vi "BuildCustomDashBoardData.vi"   [LabVIEW 2014]
doc: "This VI builds data and sends it back to the dashboard PC program. By default it sends back the raw values for the first analog, digital, and solenoid module. Modify it to send back the data you want to view. Consider adding higher level data to the Dashboard Datatype.ctl and to this VI. Then update the Dashboard to display the data however you like.\n\nThis software is licensed. Open the labview\\readme\\WPI Robotics Library Open Source License.txt file for more information."
uses:
  <vilib>/Rock Robotics/WPI/DriverStation/WPI_DriverStationRobotMode2.ctl
  typedefs/dashboard/DashboardEnable.ctl
  <vilib>/Rock Robotics/SystemInterfaces/Typedef/FPGA_TypedefDigitalModule.ctl
  typedefs/fg_getset.ctl
  <vilib>/Rock Robotics/WPI/AnalogModule/WPI_AnalogModuleDevStatus.ctl
  <vilib>/Rock Robotics/SystemInterfaces/Typedef/FPGA_TypedefAnalogModule.ctl
  <vilib>/Rock Robotics/SystemInterfaces/AI/FPGA_AIChannel.ctl
  <vilib>/Rock Robotics/WPI/Solenoid/WPI_SolenoidDevRef.ctl
  <vilib>/Rock Robotics/WPI/Solenoid/WPI_SolenoidChannel.ctl
  <vilib>/Rock Robotics/WPI/DriverStation/WPI_DriverStationDigitalData.ctl
  <vilib>/Rock Robotics/SystemInterfaces/DIO/FPGA_DIOPWMChannel.ctl
  <vilib>/Rock Robotics/Network Tables/NT Write String Array.vi
  <vilib>/Rock Robotics/WPI/Compressor/WPI_CompressorGetSetRefNum.vi
  global variables/safeties.vi
  <vilib>/Rock Robotics/WPI/Solenoid/Deprecated/WPI_SolenoidGetBool.vi
  <vilib>/Rock Robotics/SystemInterfaces/System/FPGA_SystemGet.vi
  global variables/devrefs.vi
  global variables/state machine.vi
  typedefs/dashboard/misc dash data.ctl
  typedefs/test/test controls.ctl
  global variables/vision.vi
  typedefs/state machine/performance data.ctl
panel:
  # "Generate Dashboard Data and Send it"
  # "Note: Test code calls some dashboard data, which is gotten there not here"
types:
  T1 = typedef "WPI_AnalogModuleDevStatus.ctl" = cluster{"DevStatus":errorcluster, "Controller":T2}
  T2 = typedef "FPGA_TypedefAnalogModule.ctl" = enum16{"Controller 1"}
  T3 = typedef "FPGA_AIChannel.ctl" = enum8{"AI 0", "AI 1", "AI 2", "AI 3", "AI MXP 0", "AI MXP 1", "AI MXP 2", "AI MXP 3", "Invalid"}
  T4 = typedef "FPGA_TypedefDigitalModule.ctl" = enum16{"Controller 1"}
  T5 = typedef "WPI_DriverStationDigitalData.ctl" = cluster{"Relay Fwd":u8, "Relay Rev":u8, "GPIO":u16, "GPIO_OE":u16, "PWM":cluster{"PWM[0]":u8, "PWM[1]":u8, "PWM[2]":u8, "PWM[3]":u8, "PWM[4]":u8, "PWM[5]":u8, "PWM[6]":u8, "PWM[7]":u8, "PWM[8]":u8, "PWM[9]":u8, "PWM[10]":u8, "PWM[11]":u8, "PWM[12]":u8, "PWM[13]":u8, "PWM[14]":u8, "PWM[15]":u8, "PWM[16]":u8, "PWM[17]":u8, "PWM[18]":u8, "PWM[19]":u8}}
  T6 = typedef "FPGA_DIOPWMChannel.ctl" = enum8{"PWM 0", "PWM 1", "PWM 2", "PWM 3", "PWM 4", "PWM 5", "PWM 6", "PWM 7", "PWM 8", "PWM 9", "PWM MXP 0", "PWM MXP 1", "PWM MXP 2", "PWM MXP 3", "PWM MXP 4", "PWM MXP 5", "PWM MXP 6", "PWM MXP 7", "PWM MXP 8", "PWM MXP 9", "Invalid"}
  T7 = typedef "WPI_SolenoidChannel.ctl" = enum8{"Solenoid 0", "Solenoid 1", "Solenoid 2", "Solenoid 3", "Solenoid 4", "Solenoid 5", "Solenoid 6", "Solenoid 7", "Invalid"}
  T8 = typedef "WPI_SolenoidDevRef.ctl" = cluster{"DevStatus":errorcluster, "Pneumatics Control Module":u8, "Forward Solenoid Channel":T7, "Reverse Solenoid Channel":T7}
  T9 = typedef "misc dash data.ctl" = cluster{"Performance":T10, "Vision":cluster{"distance":dbl}, "Enabled?":bool}
  T10 = typedef "performance data.ctl" = cluster{"Vision mSPI":u32, "Main mSPI":u32, "Dash mSPI":u32}
  T11 = typedef "fg_getset.ctl" = enum16{"Get", "Set"}
  T12 = typedef "WPI_DriverStationRobotMode2.ctl" = enum16{"Autonomous Disabled", "Autonomous Enabled", "Teleop Disabled", "Teleop Enabled", "Disconnected", "Finish", "Test Disabled", "Test Enabled", "Emergency Stopped"}
  T13 = typedef "DashboardEnable.ctl" = cluster{"Analog I/O":bool[], "Digital I/O":bool, "Solenoids":bool}
  T14 = typedef "subStates.ctl" = enum16{"null", "wait", "driver control", "auto", "manual override", "hold position", "rotate", "test", "end"}
  T15 = typedef "FPGA_DIODevRef.ctl" = cluster{"DevStatus":errorcluster, "Controller":T4}
  T16 = cluster{"[0]":u16, "[1]":u16, "[2]":u16, "[3]":u16, "[4]":u16, "[5]":u16, "[6]":u16, "[7]":u16, "[8]":u16, "[9]":u16}
  T17 = typedef "WPI_EncoderDevRef.ctl" = cluster{"DevStatus":errorcluster, "EncoderIndex":T18, "CounterIndex":T19, "DistancePerCount":dbl, "Decoding Type":T20}
  T18 = typedef "FPGA_EncoderIdx.ctl" = enum8{"Enc 0", "Enc 1", "Enc 2", "Enc 3", "Enc 4", "Enc 5", "Enc 6", "Enc 7", "Invalid"}
  T19 = typedef "FPGA_CounterCtrSystemIndex.ctl" = enum8{"Ctr 0", "Ctr 1", "Ctr 2", "Ctr 3", "Ctr 4", "Ctr 5", "Ctr 6", "Ctr 7", "Invalid"}
  T20 = typedef "WPI_EncoderType.ctl" = enum16{"1x", "2x", "4x"}
  T21 = typedef "WPI_CompressorDevRef.ctl" = cluster{"DevStatus":errorcluster, "Pneumatics Control Module":u8}
  T22 = typedef "WPI_MotorControlDeviceRef.ctl" = cluster{"DeviceStatus":errorcluster, "Type":T23, "PWM":cluster{"Controller":T4, "PWM Channel":T6, "DeadBand":T24}, "CAN":cluster{"Device Number":u8, "Control Mode":T25, "Semaphore":T26, "Max Vout":dbl, "TalonSRX Control Mode":T27}, "Invert":bool, "TransformRef":T28, "InvTransformRef":T28}
  T23 = typedef "WPI_MotorControlType.ctl" = enum16{"PWM", "CAN", "CANTalonSRX"}
  T24 = typedef "WPI_PWMDeadband.ctl" = cluster{"Name":string, "maxPositivePwm":i32, "minPositivePwm":i32, "centerPwm":i32, "maxNegativePwm":i32, "minNegativePwm":i32, "angularRange":u16}
  T25 = typedef "WPI_CANJaguar_ControlMode.ctl" = enum8{"Percent VBus", "Current", "Speed", "Position", "Voltage"}
  T26 = typedef "Semaphore RefNum" = refnum<k1>
  T27 = typedef "WPI_CANTalonSRX_APIControlMode.ctl" = enum8{"Percent VBus", "Speed", "Position", "Slave", "Unchanged / Invalid"}
  T28 = typedef "WPI_PWMTransform_ConPane.ctl" = refnum<vi>
  T29 = typedef "WPI_GyroDevRef.ctl" = cluster{"DevStatus":errorcluster, "Analog Module":T2, "Analog Channel":T3, "Offset":dbl, "Gain (VoltsPerDegree/Second)":dbl}
  T30 = typedef "singleUseSubstate.ctl" = enum16{"null", "wait", "extend left", "retract left", "extend right", "retract right", "end"}
  T31 = typedef "h-drive teleop safety data.ctl" = cluster{"Back Left Encoder Failure":bool, "Back Left No Rate Read":bool, "Back Right Encoder Failure":bool, "Back Right No Rate Read":bool, "Front Left Encoder Failure":bool, "Front Left No Rate Read":bool, "Front Right Encoder Failure":bool, "Front Right No Rate Read":bool, "No Gyro Rate Read":bool, "Gyro Failure":bool}
  T32 = typedef "test controls.ctl" = cluster{"Button":bool, "Switch":bool, "Slider":dbl}
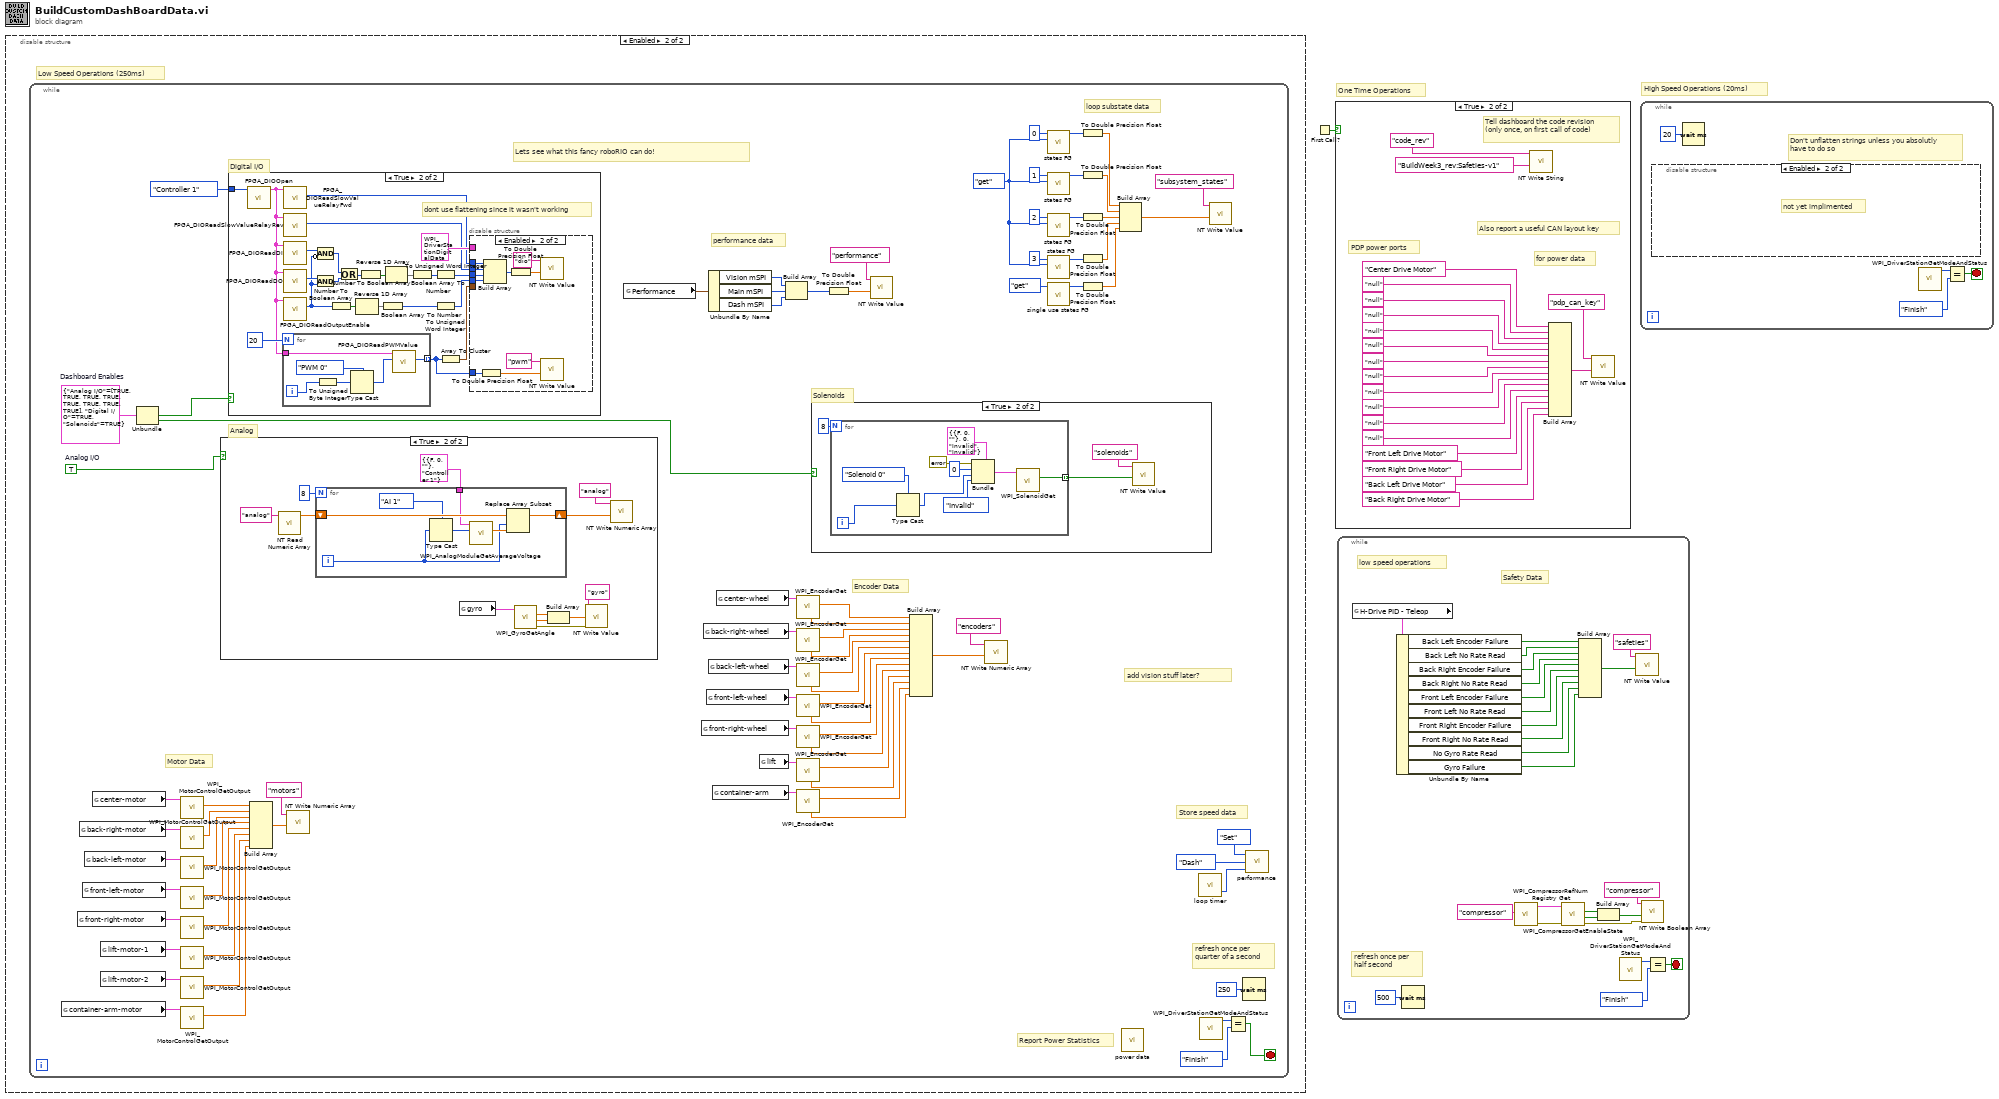
[diagram p0: block diagram]
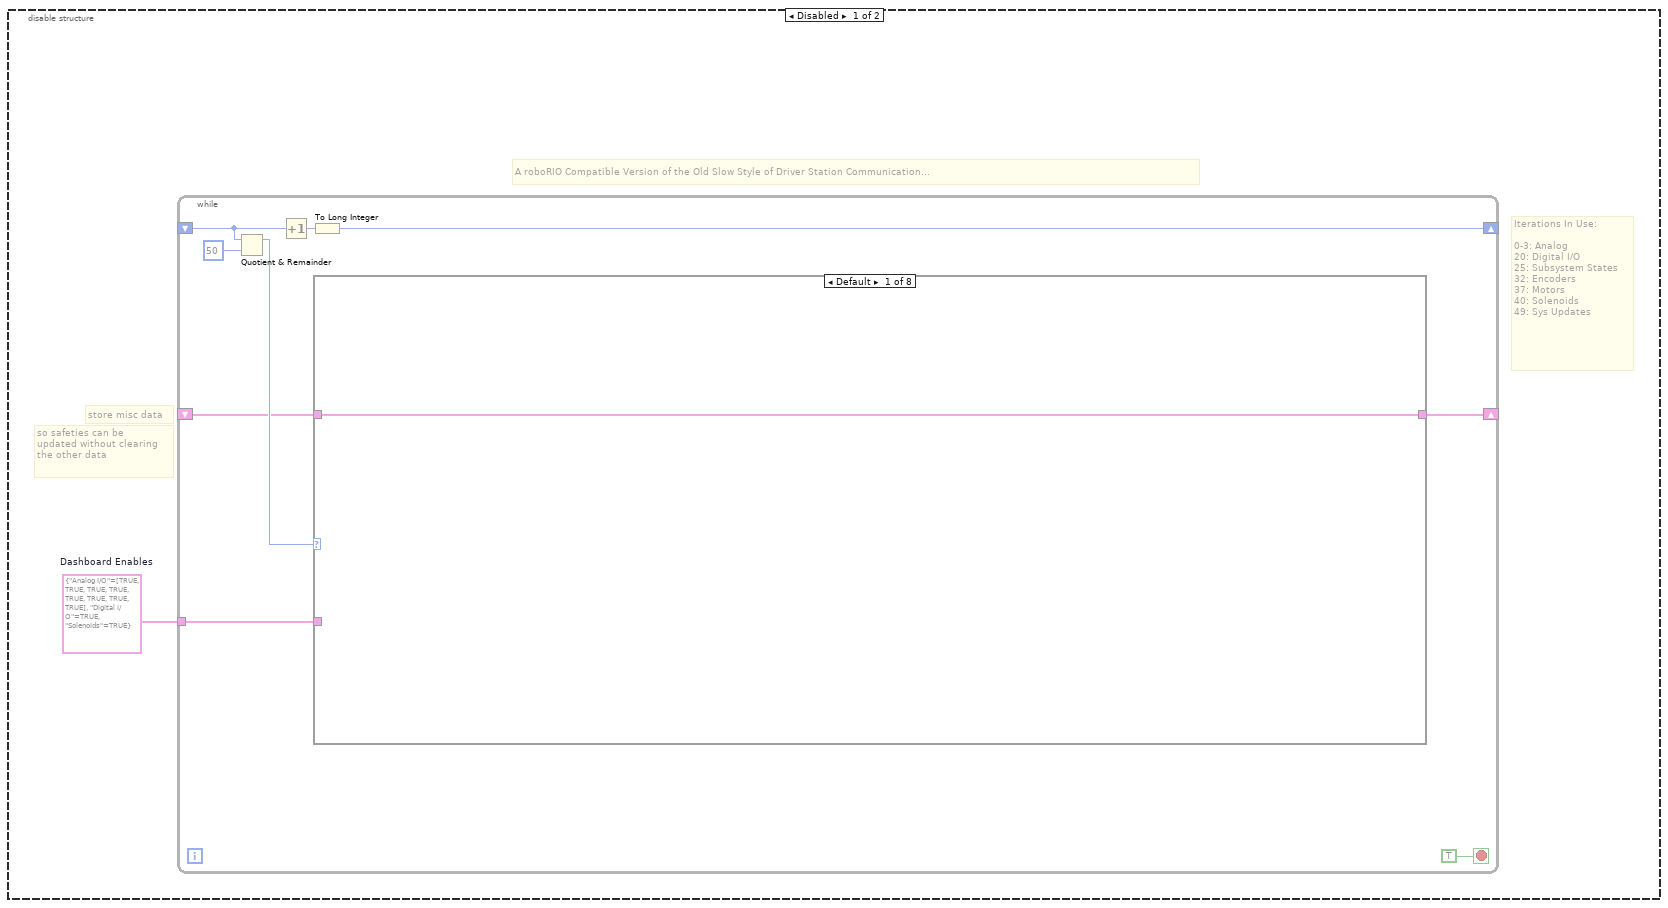
[diagram p2: hidden frame]
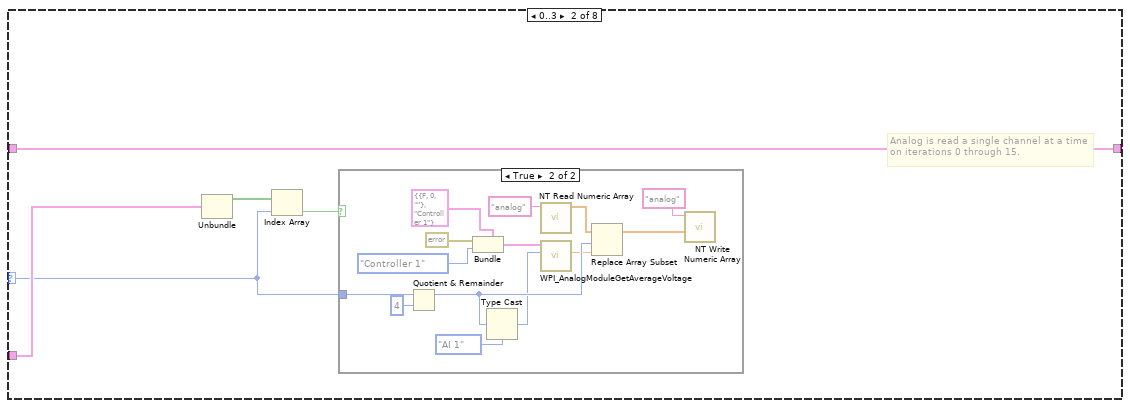
[diagram p3: hidden frame]
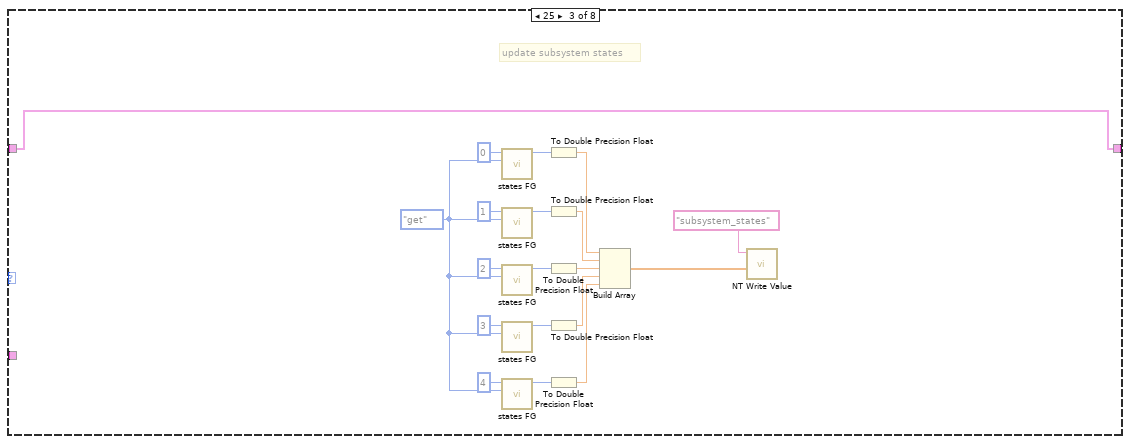
[diagram p5: hidden frame]
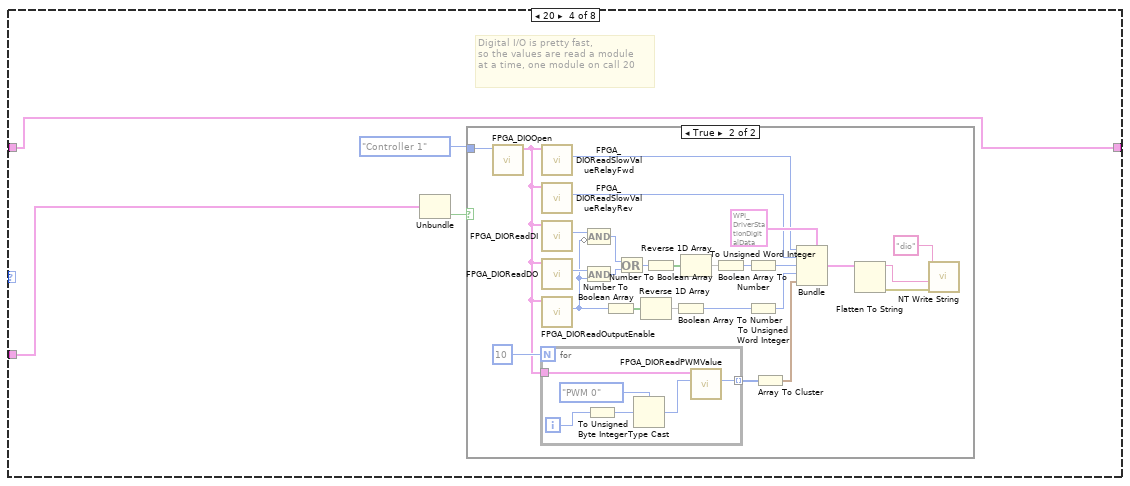
[diagram p6: hidden frame]
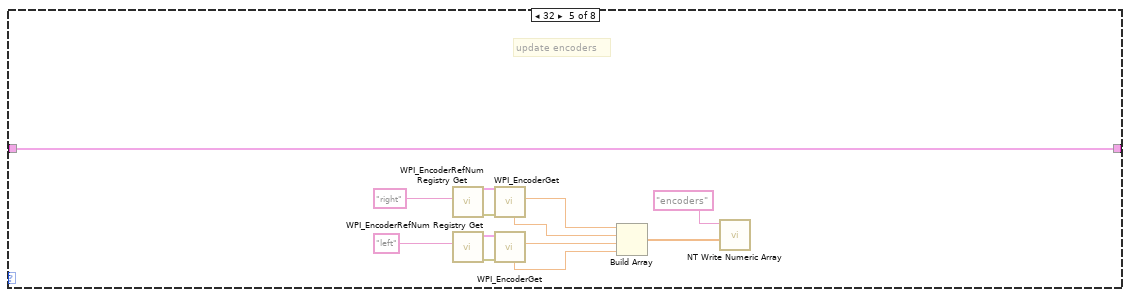
[diagram p8: hidden frame]
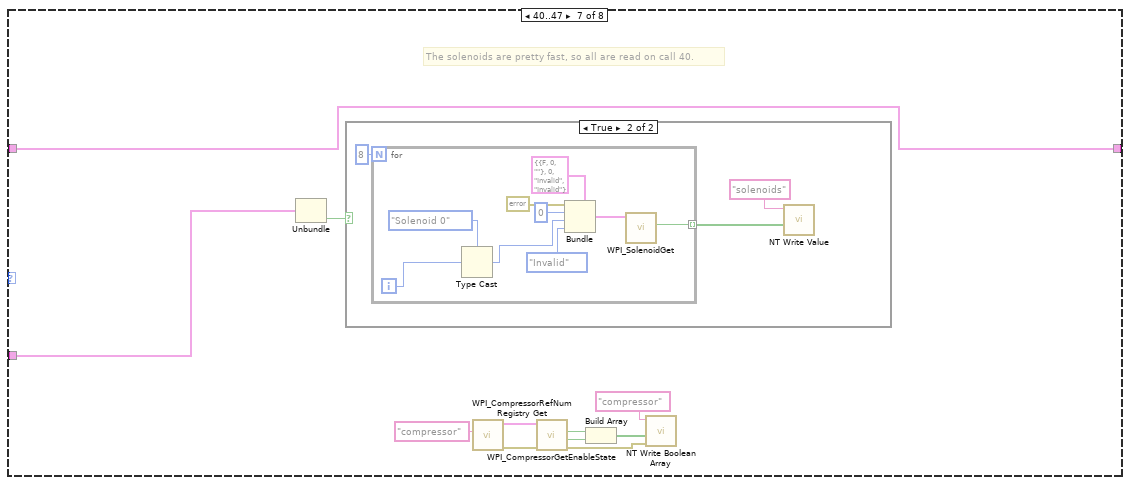
[diagram p10: hidden frame]
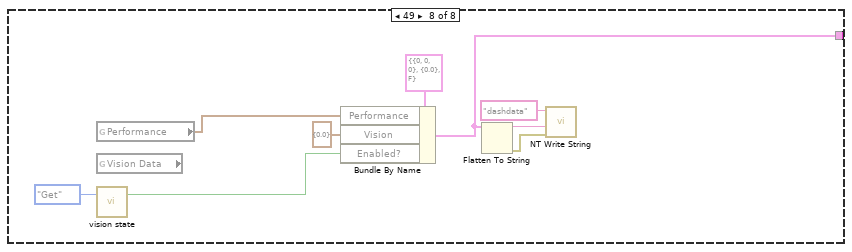
[diagram p12: hidden frame]
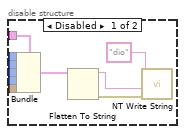
[diagram p15: hidden frame]
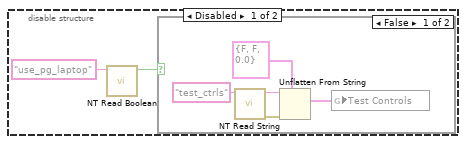
[diagram p17: hidden frame]
diagram:
  # "One Time Operations"
  # "High Speed Operations (20ms)"
  n1 = disable-structure shown="Enabled" {
    frame Disabled {
      w2 = T13 {"Analog I/O"=[TRUE, TRUE, TRUE, TRUE, TRUE, TRUE, TRUE, TRUE], "Digital I/O"=TRUE, "Solenoids"=TRUE}  # Dashboard Enables
      # "A roboRIO Compatible Version of the Old Slow Style of Driver Station Communication..."
      # "so safeties can be\nupdated without clearing\nthe other data"
      # "store misc data"
      # "Iterations In Use:\n\n0-3: Analog\n20: Digital I/O \n25: Subsystem States\n32: Encoders\n37: Motors\n40: Solenoids\n49: Sys Updates"
      n2 = while {
        shift-right: [w8] -> _
        shift-left: _ -> [w9]
        tunnel: w2 -> [w6]
        shift-right: [w4] -> _
        shift-left: _ -> [w3]
        stop <- TRUE stop-if-true
        n3 = Quotient & Remainder(x=w9, y=50) -> (x-y*floor(x/y)=w5:i32)  [unwired: 1 out]
        n4 = Increment(x=w9) -> (x+1=w10:i32)
        n5 = To Long Integer(number=w10) -> (32bit integer=w8:i32)
        n6 = case shown="Default" w5 {
          selector: w5 -> [_ w16 _ _ _ _ _ _]
          tunnel: w6 -> [_ w17 _ w54 _ _ w111 _]
          tunnel: [w12 w14 w33 w51 w89 w100 w102 w127] -> w4
          tunnel: w3 -> [w12 w14 w33 w51 w89 w100 w102 _]
          frame Default {
          }
          frame 0..3 {
            # "Analog is read a single channel at a time\non iterations 0 through 15."
            n7 = Unbundle(w17) -> ("Analog I/O"=w13:bool[])  [unwired: 2 out]
            n8 = Index Array(array=w13, index=w16) -> (element=w15:bool)
            n9 = case shown="True" w15 {
              tunnel: w16 -> [_ w29]
              frame False {
              }
              frame True {
                n10 = Quotient & Remainder(x=w29, y=4) -> (x-y*floor(x/y)=w23:i32)  [unwired: 1 out]
                n11 = Bundle(cluster=T1 {"DevStatus"={"status"=FALSE, "code"=0, "source"=""}, "Controller"=enum."Controller 1"} ("AnalogModuleDevStatus"), "DevStatus"=errorcluster {"status"=FALSE, "code"=0, "source"=""}, "Controller"=FPGA_TypedefAnalogModule."Controller 1") -> (w20:T1)
                n12 = Type Cast(type=FPGA_AIChannel."AI 1" ("Channel"), x=w23) -> (*(type *) &x=w22:T3)
                n13 = call <vilib>:"NT Read Numeric Array.vi"("Name"="analog") -> ("Numeric Array"=w27:dbl[])  [unwired: 9 in, 1 out]
                n14 = call <vilib>:"WPI_AnalogModuleGetAverageVoltage.vi"("Channel"=w22, "AnalogModuleDevStatus"=w20) -> ("Average Voltage"=w18:dbl)  [unwired: 1 in, 8 out]
                n15 = Replace Array Subset(array=w27, new element=w18, index=w23) -> (w25:dbl[])
                n16 = call <vilib>:"NT Write Numeric Array.vi"("Numeric Array"=w25, "Name"="analog") -> ()  [unwired: 9 in, 1 out]
              }
            }
          }
          frame 25 {
            w45 = enum16{"set", "get"}."get" ("menu (get)")
            # "update subsystem states"
            n17 = call "states FG.vi"("menu (get)"=w45, "Loop ID"=0) -> ("subState out"=w42:T14)  [unwired: 6 in, 3 out]
            n18 = call "states FG.vi"("menu (get)"=w45, "Loop ID"=1) -> ("subState out"=w43:T14)  [unwired: 6 in, 3 out]
            n19 = call "states FG.vi"("menu (get)"=w45, "Loop ID"=2) -> ("subState out"=w44:T14)  [unwired: 6 in, 3 out]
            n20 = call "states FG.vi"("menu (get)"=w45, "Loop ID"=3) -> ("subState out"=w41:T14)  [unwired: 6 in, 3 out]
            n21 = call "states FG.vi"("menu (get)"=w45, "Loop ID"=4) -> ("subState out"=w40:T14)  [unwired: 6 in, 3 out]
            n22 = To Double Precision Float(number=w42) -> (double precision float=w38:dbl)
            n23 = To Double Precision Float(number=w43) -> (double precision float=w37:dbl)
            n24 = To Double Precision Float(number=w44) -> (double precision float=w36:dbl)
            n25 = To Double Precision Float(number=w41) -> (double precision float=w35:dbl)
            n26 = To Double Precision Float(number=w40) -> (double precision float=w34:dbl)
            n27 = Build Array(w38, w37, w36, w35, w34) -> (w32:dbl[])
            n28 = call-poly <vilib>:"NT Write Value.vi"("Numeric Array"=w32, "Name"="subsystem_states") -> ()  [unwired: 9 in, 1 out]
          }
          frame 20 {
            # "Digital I/O is pretty fast,\nso the values are read a module\nat a time, one module on call 20"
            n29 = Unbundle(w54) -> ("Solenoids"=w52:bool)  [unwired: 2 out]
            n30 = case shown="True" w52 {
              tunnel: FPGA_TypedefDigitalModule."Controller 1" ("Module (Module 1)") -> [_ w61]
              frame False {
              }
              frame True {
                n31 = call <vilib>:"FPGA_DIOOpen.vi"("Controller"=w61) -> ("DIODeviceRef"=w77:T15)  [unwired: 1 in, 9 out]
                n32 = for {
                  N: 10 -> [_]
                  tunnel: w77 -> [w86]
                  tunnel: [w84] -> w78 mode=indexing
                  i -> [w85]
                  n33 = To Unsigned Byte Integer(number=w85) -> (unsigned 8bit integer=w83:u8)
                  n34 = Type Cast(type=FPGA_DIOPWMChannel."PWM 0" ("PWMChannel"), x=w83) -> (*(type *) &x=w81:T6)
                  n35 = call <vilib>:"FPGA_DIOReadPWMValue.vi"("PWMChannel"=w81, "DIODeviceRef In"=w86) -> ("PWMValue"=w84:u16)  [unwired: 1 in, 8 out]
                }
                n36 = call <vilib>:"FPGA_DIOReadSlowValueRelayFwd.vi"("DIODeviceRef In"=w77) -> ("Relay Forward"=w70:u8)  [unwired: 1 in, 9 out]
                n37 = call <vilib>:"FPGA_DIOReadSlowValueRelayRev.vi"("DIODeviceRef In"=w77) -> ("Relay Reverse"=w71:u8)  [unwired: 1 in, 9 out]
                n38 = call <vilib>:"FPGA_DIOReadDI.vi"("DIODeviceRef In"=w77) -> ("DI"=w75:u32)  [unwired: 1 in, 9 out]
                n39 = call <vilib>:"FPGA_DIOReadDO.vi"("DIODeviceRef In"=w77) -> ("DO"=w74:u32)  [unwired: 1 in, 9 out]
                n40 = call <vilib>:"FPGA_DIOReadOutputEnable.vi"("DIODeviceRef In"=w77) -> ("OutputEnable"=w65:u32)  [unwired: 1 in, 9 out]
                n41 = And(x=w74, y=w65) -> (x .and. y?=w73:u32)
                n42 = Compound Arithmetic op=AND(w75, invert w65) -> (w72:u32)
                n43 = Number To Boolean Array(number=w65) -> (Boolean array=w67:bool[])
                n44 = Or(x=w72, y=w73) -> (x .or. y?=w63:u32)
                n45 = Reverse 1D Array(array=w67) -> (reversed array=w66:bool[])
                n46 = Number To Boolean Array(number=w63) -> (Boolean array=w68:bool[])
                n47 = Boolean Array To Number(Boolean array=w66) -> (number=w64:u32)
                n48 = Reverse 1D Array(array=w68) -> (reversed array=w69:bool[])
                n49 = Boolean Array To Number(Boolean array=w69) -> (number=w62:u32)
                n50 = To Unsigned Word Integer(number=w62) -> (unsigned 16bit integer=w55:u16)
                n51 = To Unsigned Word Integer(number=w64) -> (unsigned 16bit integer=w56:u16)
                n52 = Array To Cluster(array=w78) -> (cluster=w76:T16)
                n53 = Bundle(cluster=T5 {"Relay Fwd"=0, "Relay Rev"=0, "GPIO"=0, "GPIO_OE"=0, "PWM"={"PWM[0]"=0, "PWM[1]"=0, "PWM[2]"=0, "PWM[3]"=0, "PWM[4]"=0, "PWM[5]"=0, "PWM[6]"=0, "PWM[7]"=0, "PWM[8]"=0, "PWM[9]"=0, "PWM[10]"=0, "PWM[11]"=0, "PWM[12]"=0, "PWM[13]"=0, "PWM[14]"=0, "PWM[15]"=0, "PWM[16]"=0, "PWM[17]"=0, "PWM[18]"=0, "PWM[19]"=0}} ("DigitalModule"), "Relay Fwd"=w70, "Relay Rev"=w71, "GPIO"=w55, "GPIO_OE"=w56, "PWM"=w76) -> (w60:T5)
                n54 = Flatten To String(anything=w60) -> (data string=w58:string, error out=w59:errorcluster)  [unwired: 1 in, 3 out]
                n55 = call <vilib>:"NT Write String.vi"("error in"=w59, "String"=w58, "Name"="dio") -> ()  [unwired: 8 in, 1 out]
              }
            }
          }
          frame 32 {
            # "update encoders"
            n56 = call <vilib>:"WPI_EncoderRefNum Registry Get.vi"("refnum name"="right") -> ("error out"=w97:errorcluster, "EncoderDevRef"=w96:T17)  [unwired: 9 in]
            n57 = call <vilib>:"WPI_EncoderRefNum Registry Get.vi"("refnum name"="left") -> ("error out"=w94:errorcluster, "EncoderDevRef"=w95:T17)  [unwired: 9 in]
            n58 = call <vilib>:"WPI_EncoderGet.vi"("error in (no error)"=w97, "EncoderDevRef"=w96) -> ("Distance"=w93:dbl, "Rate"=w88:dbl)  [unwired: 4 in, 4 out]
            n59 = call <vilib>:"WPI_EncoderGet.vi"("error in (no error)"=w94, "EncoderDevRef"=w95) -> ("Distance"=w92:dbl, "Rate"=w91:dbl)  [unwired: 4 in, 4 out]
            n60 = Build Array(w93, w88, w92, w91) -> (w90:dbl[])
            n61 = call <vilib>:"NT Write Numeric Array.vi"("Numeric Array"=w90, "Name"="encoders") -> ()  [unwired: 9 in, 1 out]
          }
          frame 37 {
            # "update motor array"
          }
          frame 40..47 {
            # "The solenoids are pretty fast, so all are read on call 40."
            n62 = Unbundle(w111) -> ("Solenoids"=w101:bool)  [unwired: 2 out]
            n63 = case shown="True" w101 {
              frame False {
              }
              frame True {
                n64 = for {
                  N: 8 -> [_]
                  tunnel: [w115] -> w113 mode=indexing
                  i -> [w117]
                  n65 = Type Cast(type=WPI_SolenoidChannel."Solenoid 0" ("Forward Solenoid Channel"), x=w117) -> (*(type *) &x=w116:T7)
                  n66 = Bundle(cluster=T8 {"DevStatus"={"status"=FALSE, "code"=0, "source"=""}, "Pneumatics Control Module"=0, "Forward Solenoid Channel"=enum."Invalid", "Reverse Solenoid Channel"=enum."Invalid"} ("SolenoidDevRef"), "DevStatus"=errorcluster {"status"=FALSE, "code"=0, "source"=""}, "Pneumatics Control Module"=u8 0, "Forward Solenoid Channel"=w116, "Reverse Solenoid Channel"=WPI_SolenoidChannel."Invalid") -> (w122:T8)
                  n67 = call-poly <vilib>:"WPI_SolenoidGet.vi"("SolenoidDevRef"=w122) -> ("Value"=w115:bool)  [unwired: 8 in, 2 out]
                }
                n68 = call-poly <vilib>:"NT Write Value.vi"("Boolean Array"=w113, "Name"="solenoids") -> ()  [unwired: 9 in, 1 out]
              }
            }
            n69 = call <vilib>:"WPI_CompressorRefNum Registry Get.vi"("refnum name"="compressor") -> ("error out"=w107:errorcluster, "CompressorDevRef"=w108:T21)  [unwired: 9 in]
            n70 = call <vilib>:"WPI_CompressorGetEnableState.vi"("error in (no error)"=w107, "CompressorDevRef"=w108) -> ("error out"=w103:errorcluster, "Compressor Running"=w105:bool, "Enabled"=w106:bool)  [unwired: 6 in, 1 out]
            n71 = Build Array(w106, w105) -> (w104:bool[])
            n72 = call <vilib>:"NT Write Boolean Array.vi"("error in"=w103, "Boolean Array"=w104, "Name"="compressor") -> ()  [unwired: 8 in, 1 out]
          }
          frame 49 {
            n73 = global read "state machine.vi" "Performance"() -> (w124:T10)
            n74 = global read "vision.vi" "Vision Data"() -> ()  [unwired: 1 out]
            n75 = call "vision state.vi"("Menu"=fg_getset."Get") -> ("Enabled?"=w126:bool)  [unwired: 1 in, 1 out]
            n76 = Bundle By Name(cluster=T9 {"Performance"={"Vision mSPI"=0, "Main mSPI"=0, "Dash mSPI"=0}, "Vision"={"distance"=0.0}, "Enabled?"=FALSE}, "Performance"=w124, "Vision"=cluster{"distance":dbl} {"distance"=0.0}, "Enabled?"=w126) -> (w127:T9)
            n77 = Flatten To String(anything=w127) -> (data string=w130:string, error out=w128:errorcluster)  [unwired: 1 in, 3 out]
            n78 = call <vilib>:"NT Write String.vi"("error in"=w128, "String"=w130, "Name"="dashdata") -> ()  [unwired: 8 in, 1 out]
          }
        }
      }
    }
    frame Enabled {
      # "Low Speed Operations (250ms)"
      n79 = while {
        stop <- w191 stop-if-true
        w182 = TRUE  # Analog I/O
        w205 = enum16{"set", "get"}."get" ("menu (get)")
        w210 = T13 {"Analog I/O"=[TRUE, TRUE, TRUE, TRUE, TRUE, TRUE, TRUE, TRUE], "Digital I/O"=TRUE, "Solenoids"=TRUE}  # Dashboard Enables
        # "Encoder Data"
        # "Motor Data"
        # "loop substate data"
        # "performance data"
        # "add vision stuff later?"
        # "Report Power Statistics"
        # "Store speed data"
        # "refresh once per\nquarter of a second"
        # "Solenoids"
        # "Digital I/O"
        # "Analog"
        # "Lets see what this fancy roboRIO can do!"
        n80 = global read "devrefs.vi" "container-arm-motor"() -> (w150:T22)
        n81 = global read "devrefs.vi" "front-right-motor"() -> (w154:T22)
        n82 = global read "devrefs.vi" "back-right-motor"() -> (w157:T22)
        n83 = global read "devrefs.vi" "front-left-motor"() -> (w155:T22)
        n84 = global read "devrefs.vi" "back-left-motor"() -> (w156:T22)
        n85 = global read "devrefs.vi" "center-motor"() -> (w153:T22)
        n86 = global read "devrefs.vi" "lift-motor-1"() -> (w152:T22)
        n87 = global read "devrefs.vi" "lift-motor-2"() -> (w151:T22)
        n88 = Unbundle(w210) -> ("Digital I/O"=w195:bool, "Solenoids"=w181:bool)  [unwired: 1 out]
        n89 = call <vilib>:"WPI_MotorControlGetOutput.vi"("MotorControlDevRef"=w153) -> ("Output"=w149:dbl)  [unwired: 8 in, 2 out]
        n90 = call <vilib>:"WPI_MotorControlGetOutput.vi"("MotorControlDevRef"=w157) -> ("Output"=w148:dbl)  [unwired: 8 in, 2 out]
        n91 = call <vilib>:"WPI_MotorControlGetOutput.vi"("MotorControlDevRef"=w156) -> ("Output"=w147:dbl)  [unwired: 8 in, 2 out]
        n92 = call <vilib>:"WPI_MotorControlGetOutput.vi"("MotorControlDevRef"=w155) -> ("Output"=w146:dbl)  [unwired: 8 in, 2 out]
        n93 = call <vilib>:"WPI_MotorControlGetOutput.vi"("MotorControlDevRef"=w154) -> ("Output"=w145:dbl)  [unwired: 8 in, 2 out]
        n94 = call <vilib>:"WPI_MotorControlGetOutput.vi"("MotorControlDevRef"=w152) -> ("Output"=w144:dbl)  [unwired: 8 in, 2 out]
        n95 = call <vilib>:"WPI_MotorControlGetOutput.vi"("MotorControlDevRef"=w151) -> ("Output"=w143:dbl)  [unwired: 8 in, 2 out]
        n96 = call <vilib>:"WPI_MotorControlGetOutput.vi"("MotorControlDevRef"=w150) -> ("Output"=w142:dbl)  [unwired: 8 in, 2 out]
        n97 = case shown="True" w182 {
          frame False {
          }
          frame True {
            n98 = call <vilib>:"NT Read Numeric Array.vi"("Name"="analog") -> ("Numeric Array"=w281:dbl[])  [unwired: 9 in, 1 out]
            n99 = for {
              N: 8 -> [_]
              tunnel: T1 {"DevStatus"={"status"=FALSE, "code"=0, "source"=""}, "Controller"=enum."Controller 1"} ("AnalogModuleDevStatus") -> [w284]
              shift-right: [w288] -> w280
              shift-left: w281 -> [w289]
              i -> [w283]
              n100 = Type Cast(type=FPGA_AIChannel."AI 1" ("Channel"), x=w283) -> (*(type *) &x=w286:T3)
              n101 = call <vilib>:"WPI_AnalogModuleGetAverageVoltage.vi"("Channel"=w286, "AnalogModuleDevStatus"=w284) -> ("Average Voltage"=w285:dbl)  [unwired: 1 in, 8 out]
              n102 = Replace Array Subset(array=w289, new element=w285, index=w283) -> (w288:dbl[])
            }
            n103 = global read "devrefs.vi" "gyro"() -> (w275:T29)
            n104 = call <vilib>:"WPI_GyroGetAngle.vi"("GyroDevRef"=w275) -> ("error out"=w276:errorcluster, "Angular Rate"=w273:dbl, "Angle"=w274:dbl)  [unwired: 7 in, 1 out]
            n105 = Build Array(w274, w273) -> (w272:dbl[])
            n106 = call-poly <vilib>:"NT Write Value.vi"("error in"=w276, "Numeric Array"=w272, "Name"="gyro") -> ()  [unwired: 8 in, 1 out]
            n107 = call <vilib>:"NT Write Numeric Array.vi"("Numeric Array"=w280, "Name"="analog") -> ()  [unwired: 9 in, 1 out]
          }
        }
        n108 = case shown="True" w195 {
          tunnel: FPGA_TypedefDigitalModule."Controller 1" ("Module (Module 1)") -> [_ w226]
          frame False {
          }
          frame True {
            # "dont use flattening since it wasn't working"
            n109 = call <vilib>:"FPGA_DIOOpen.vi"("Controller"=w226) -> ("DIODeviceRef"=w242:T15)  [unwired: 1 in, 9 out]
            n110 = for {
              N: 20 -> [_]
              tunnel: w242 -> [w270]
              tunnel: [w268] -> w223 mode=indexing
              i -> [w269]
              n111 = To Unsigned Byte Integer(number=w269) -> (unsigned 8bit integer=w267:u8)
              n112 = Type Cast(type=FPGA_DIOPWMChannel."PWM 0" ("PWMChannel"), x=w267) -> (*(type *) &x=w265:T6)
              n113 = call <vilib>:"FPGA_DIOReadPWMValue.vi"("PWMChannel"=w265, "DIODeviceRef In"=w270) -> ("PWMValue"=w268:u16)  [unwired: 1 in, 8 out]
            }
            n114 = call <vilib>:"FPGA_DIOReadSlowValueRelayFwd.vi"("DIODeviceRef In"=w242) -> ("Relay Forward"=w235:u8)  [unwired: 1 in, 9 out]
            n115 = call <vilib>:"FPGA_DIOReadSlowValueRelayRev.vi"("DIODeviceRef In"=w242) -> ("Relay Reverse"=w236:u8)  [unwired: 1 in, 9 out]
            n116 = call <vilib>:"FPGA_DIOReadDI.vi"("DIODeviceRef In"=w242) -> ("DI"=w240:u32)  [unwired: 1 in, 9 out]
            n117 = call <vilib>:"FPGA_DIOReadDO.vi"("DIODeviceRef In"=w242) -> ("DO"=w239:u32)  [unwired: 1 in, 9 out]
            n118 = call <vilib>:"FPGA_DIOReadOutputEnable.vi"("DIODeviceRef In"=w242) -> ("OutputEnable"=w230:u32)  [unwired: 1 in, 9 out]
            n119 = And(x=w239, y=w230) -> (x .and. y?=w238:u32)
            n120 = Compound Arithmetic op=AND(w240, invert w230) -> (w237:u32)
            n121 = Number To Boolean Array(number=w230) -> (Boolean array=w232:bool[])
            n122 = Or(x=w237, y=w238) -> (x .or. y?=w228:u32)
            n123 = Reverse 1D Array(array=w232) -> (reversed array=w231:bool[])
            n124 = Number To Boolean Array(number=w228) -> (Boolean array=w233:bool[])
            n125 = Boolean Array To Number(Boolean array=w231) -> (number=w229:u32)
            n126 = Reverse 1D Array(array=w233) -> (reversed array=w234:bool[])
            n127 = Boolean Array To Number(Boolean array=w234) -> (number=w227:u32)
            n128 = To Unsigned Word Integer(number=w227) -> (unsigned 16bit integer=w224:u16)
            n129 = To Unsigned Word Integer(number=w229) -> (unsigned 16bit integer=w225:u16)
            n130 = Array To Cluster(array=w223) -> (cluster=w241:T16)
            n131 = disable-structure shown="Enabled" {
              disable-tunnel: T5 {"Relay Fwd"=0, "Relay Rev"=0, "GPIO"=0, "GPIO_OE"=0, "PWM"={"PWM[0]"=0, "PWM[1]"=0, "PWM[2]"=0, "PWM[3]"=0, "PWM[4]"=0, "PWM[5]"=0, "PWM[6]"=0, "PWM[7]"=0, "PWM[8]"=0, "PWM[9]"=0, "PWM[10]"=0, "PWM[11]"=0, "PWM[12]"=0, "PWM[13]"=0, "PWM[14]"=0, "PWM[15]"=0, "PWM[16]"=0, "PWM[17]"=0, "PWM[18]"=0, "PWM[19]"=0}} ("DigitalModule") -> [w254 _]
              disable-tunnel: w241 -> [w253 _]
              disable-tunnel: w236 -> [w252 w259]
              disable-tunnel: w235 -> [w251 w260]
              disable-tunnel: w225 -> [w246 w257]
              disable-tunnel: w224 -> [w245 w258]
              disable-tunnel: w223 -> [_ w263]
              frame Disabled {
                n132 = Bundle(cluster=w254, "Relay Fwd"=w251, "Relay Rev"=w252, "GPIO"=w245, "GPIO_OE"=w246, "PWM"=w253) -> (w250:T5)
                n133 = Flatten To String(anything=w250) -> (data string=w248:string, error out=w249:errorcluster)  [unwired: 1 in, 3 out]
                n134 = call <vilib>:"NT Write String.vi"("error in"=w249, "String"=w248, "Name"="dio") -> ()  [unwired: 8 in, 1 out]
              }
              frame Enabled {
                n135 = To Double Precision Float(number=w263) -> (double precision float=w262:dbl[])
                n136 = Build Array(w260, w259, w258, w257) -> (w256:u16[])
                n137 = To Double Precision Float(number=w256) -> (double precision float=w255:dbl[])
                n138 = call-poly <vilib>:"NT Write Value.vi"("Numeric Array"=w255, "Name"="dio") -> ()  [unwired: 9 in, 1 out]
                n139 = call-poly <vilib>:"NT Write Value.vi"("Numeric Array"=w262, "Name"="pwm") -> ()  [unwired: 9 in, 1 out]
              }
            }
          }
        }
        n140 = Build Array(w149, w148, w147, w146, w145, w144, w143, w142) -> (w140:dbl[])
        n141 = call <vilib>:"NT Write Numeric Array.vi"("Numeric Array"=w140, "Name"="motors") -> ()  [unwired: 9 in, 1 out]
        n142 = global read "state machine.vi" "Performance"() -> (w139:T10)
        n143 = global read "devrefs.vi" "front-right-wheel"() -> (w160:T17)
        n144 = global read "devrefs.vi" "back-right-wheel"() -> (w163:T17)
        n145 = global read "devrefs.vi" "front-left-wheel"() -> (w161:T17)
        n146 = Unbundle By Name(w139) -> ("Vision mSPI"=w138:u32, "Main mSPI"=w137:u32, "Dash mSPI"=w136:u32)
        n147 = global read "devrefs.vi" "back-left-wheel"() -> (w162:T17)
        n148 = global read "devrefs.vi" "container-arm"() -> (w158:T17)
        n149 = global read "devrefs.vi" "center-wheel"() -> (w164:T17)
        n150 = global read "devrefs.vi" "lift"() -> (w159:T17)
        n151 = Build Array(w138, w137, w136) -> (w135:u32[])
        n152 = call <vilib>:"WPI_EncoderGet.vi"("EncoderDevRef"=w164) -> ("Distance"=w180:dbl, "Rate"=w176:dbl)  [unwired: 5 in, 4 out]
        n153 = call <vilib>:"WPI_EncoderGet.vi"("EncoderDevRef"=w163) -> ("Distance"=w179:dbl, "Rate"=w178:dbl)  [unwired: 5 in, 4 out]
        n154 = call <vilib>:"WPI_EncoderGet.vi"("EncoderDevRef"=w162) -> ("Distance"=w174:dbl, "Rate"=w173:dbl)  [unwired: 5 in, 4 out]
        n155 = call <vilib>:"WPI_EncoderGet.vi"("EncoderDevRef"=w161) -> ("Distance"=w172:dbl, "Rate"=w171:dbl)  [unwired: 5 in, 4 out]
        n156 = call <vilib>:"WPI_EncoderGet.vi"("EncoderDevRef"=w160) -> ("Distance"=w170:dbl, "Rate"=w169:dbl)  [unwired: 5 in, 4 out]
        n157 = call <vilib>:"WPI_EncoderGet.vi"("EncoderDevRef"=w159) -> ("Distance"=w168:dbl, "Rate"=w167:dbl)  [unwired: 5 in, 4 out]
        n158 = call <vilib>:"WPI_EncoderGet.vi"("EncoderDevRef"=w158) -> ("Distance"=w166:dbl, "Rate"=w165:dbl)  [unwired: 5 in, 4 out]
        n159 = case shown="True" w181 {
          frame False {
          }
          frame True {
            n160 = for {
              N: 8 -> [_]
              tunnel: [w214] -> w212 mode=indexing
              i -> [w216]
              n161 = Type Cast(type=WPI_SolenoidChannel."Solenoid 0" ("Forward Solenoid Channel"), x=w216) -> (*(type *) &x=w215:T7)
              n162 = Bundle(cluster=T8 {"DevStatus"={"status"=FALSE, "code"=0, "source"=""}, "Pneumatics Control Module"=0, "Forward Solenoid Channel"=enum."Invalid", "Reverse Solenoid Channel"=enum."Invalid"} ("SolenoidDevRef"), "DevStatus"=errorcluster {"status"=FALSE, "code"=0, "source"=""}, "Pneumatics Control Module"=u8 0, "Forward Solenoid Channel"=w215, "Reverse Solenoid Channel"=WPI_SolenoidChannel."Invalid") -> (w221:T8)
              n163 = call-poly <vilib>:"WPI_SolenoidGet.vi"("SolenoidDevRef"=w221) -> ("Value"=w214:bool)  [unwired: 8 in, 2 out]
            }
            n164 = call-poly <vilib>:"NT Write Value.vi"("Boolean Array"=w212, "Name"="solenoids") -> ()  [unwired: 9 in, 1 out]
          }
        }
        n165 = To Double Precision Float(number=w135) -> (double precision float=w134:dbl[])
        n166 = call-poly <vilib>:"NT Write Value.vi"("Numeric Array"=w134, "Name"="performance") -> ()  [unwired: 9 in, 1 out]
        n167 = Build Array(w180, w176, w179, w178, w174, w173, w172, w171, w170, w169, w168, w167, w166, w165) -> (w177:dbl[])
        n168 = call <vilib>:"NT Write Numeric Array.vi"("Numeric Array"=w177, "Name"="encoders") -> ()  [unwired: 9 in, 1 out]
        n169 = call "states FG.vi"("menu (get)"=w205, "Loop ID"=0) -> ("subState out"=w202:T14)  [unwired: 6 in, 3 out]
        n170 = call "states FG.vi"("menu (get)"=w205, "Loop ID"=1) -> ("subState out"=w203:T14)  [unwired: 6 in, 3 out]
        n171 = call "states FG.vi"("menu (get)"=w205, "Loop ID"=2) -> ("subState out"=w204:T14)  [unwired: 6 in, 3 out]
        n172 = call "states FG.vi"("menu (get)"=w205, "Loop ID"=3) -> ("subState out"=w201:T14)  [unwired: 6 in, 3 out]
        n173 = call "single use states FG.vi"("menu (get)"=enum16{"set", "get"}."get") -> ("substate out"=w183:T30)  [unwired: 7 in, 3 out]
        n174 = To Double Precision Float(number=w202) -> (double precision float=w199:dbl)
        n175 = To Double Precision Float(number=w203) -> (double precision float=w198:dbl)
        n176 = To Double Precision Float(number=w204) -> (double precision float=w197:dbl)
        n177 = To Double Precision Float(number=w201) -> (double precision float=w185:dbl)
        n178 = To Double Precision Float(number=w183) -> (double precision float=w184:dbl)
        n179 = Build Array(w199, w198, w197, w185, w184) -> (w187:dbl[])
        n180 = call "power data.vi"() -> ()  [unwired: 12 in]
        n181 = call "loop timer.vi"() -> ("mSPI"=w188:u32)  [unwired: 1 in, 1 out]
        n182 = call <vilib>:"WPI_DriverStationGetModeAndStatus.vi"() -> ("Robot Mode"=w193:T12)  [unwired: 10 in, 1 out]
        n183 = call-poly <vilib>:"NT Write Value.vi"("Numeric Array"=w187, "Name"="subsystem_states") -> ()  [unwired: 9 in, 1 out]
        n184 = Equal?(x=w193, y=WPI_DriverStationRobotMode2."Finish") -> (x = y?=w191:bool)
        n185 = Wait (ms)(milliseconds to wait=u32 250) -> ()  [unwired: 1 out]
        n186 = call "performance.vi"("mSPI"=w188, "Loop"=enum16{"Vision", "Main", "Dash"}."Dash", "Menu"=fg_getset."Set") -> ()  [unwired: 1 out]
      }
    }
  }
  n187 = First Call?() -> (First Call?: T/F=w1:bool)
  n188 = case shown="True" w1 {
    frame False {
    }
    frame True {
      # "PDP power ports"
      # "Also report a useful CAN layout key"
      # "Tell dashboard the code revision \n(only once, on first call of code)"
      # "for power data"
      n189 = call <vilib>:"NT Write String.vi"("String"="BuildWeek3_rev:Safeties-v1", "Name"="code_rev") -> ()  [unwired: 9 in, 1 out]
      n190 = Build Array("Center Drive Motor", "null", "null", "null", "null", "null", "null", "null", "null", "null", "null", "null", "Front Left Drive Motor", "Front Right Drive Motor", "Back Left Drive Motor", "Back Right Drive Motor") -> (w302:string[])
      n191 = call-poly <vilib>:"NT Write Value.vi"("String Array"=w302, "Name"="pdp_can_key") -> ()  [unwired: 9 in, 1 out]
    }
  }
  n192 = while {
    stop <- w321 stop-if-true
    # "refresh once per\nhalf second"
    # "Safety Data"
    # "low speed operations"
    n193 = global read "safeties.vi" "H-Drive PID - Teleop"() -> (w320:T31)
    n194 = Unbundle By Name(w320) -> ("Back Left Encoder Failure"=w319:bool, "Back Left No Rate Read"=w318:bool, "Back Right Encoder Failure"=w317:bool, "Back Right No Rate Read"=w316:bool, "Front Left Encoder Failure"=w315:bool, "Front Left No Rate Read"=w314:bool, "Front Right Encoder Failure"=w313:bool, "Front Right No Rate Read"=w312:bool, "No Gyro Rate Read"=w311:bool, "Gyro Failure"=w310:bool)
    n195 = Wait (ms)(milliseconds to wait=u32 500) -> ()  [unwired: 1 out]
    n196 = call <vilib>:"WPI_CompressorRefNum Registry Get.vi"("refnum name"="compressor") -> ("error out"=w329:errorcluster, "CompressorDevRef"=w330:T21)  [unwired: 9 in]
    n197 = call <vilib>:"WPI_CompressorGetEnableState.vi"("error in (no error)"=w329, "CompressorDevRef"=w330) -> ("error out"=w325:errorcluster, "Compressor Running"=w327:bool, "Enabled"=w328:bool)  [unwired: 6 in, 1 out]
    n198 = Build Array(w319, w318, w317, w316, w315, w314, w313, w312, w311, w310) -> (w334:bool[])
    n199 = Build Array(w328, w327) -> (w326:bool[])
    n200 = call <vilib>:"WPI_DriverStationGetModeAndStatus.vi"() -> ("Robot Mode"=w322:T12)  [unwired: 10 in, 1 out]
    n201 = call-poly <vilib>:"NT Write Value.vi"("Boolean Array"=w334, "Name"="safeties") -> ()  [unwired: 9 in, 1 out]
    n202 = call <vilib>:"NT Write Boolean Array.vi"("error in"=w325, "Boolean Array"=w326, "Name"="compressor") -> ()  [unwired: 8 in, 1 out]
    n203 = Equal?(x=w322, y=WPI_DriverStationRobotMode2."Finish") -> (x = y?=w321:bool)
  }
  n204 = while {
    stop <- w336 stop-if-true
    # "Don't unflatten strings unless you absolutly\nhave to do so"
    n205 = disable-structure shown="Enabled" {
      frame Disabled {
        n206 = call <vilib>:"NT Read Boolean.vi"("Name"="use_pg_laptop") -> ("Boolean"=w340:bool)  [unwired: 9 in, 1 out]
        n207 = case shown="False" w340 {
          frame False {
            n208 = call <vilib>:"NT Read String.vi"("Name"="test_ctrls") -> ("error out"=w344:errorcluster, "String"=w343:string)  [unwired: 9 in]
            n209 = Unflatten From String(type=T32 {"Button"=FALSE, "Switch"=FALSE, "Slider"=0.0} ("Test Controls"), binary string=w343, error in (no error)=w344) -> (value=w341:T32)  [unwired: 2 in, 2 out]
            n210 = global write "state machine.vi" "Test Controls"(w341) -> ()
          }
          frame True {
          }
        }
      }
      frame Enabled {
        # "not yet implimented"
      }
    }
    n211 = Wait (ms)(milliseconds to wait=u32 20) -> ()  [unwired: 1 out]
    n212 = call <vilib>:"WPI_DriverStationGetModeAndStatus.vi"() -> ("Robot Mode"=w337:T12)  [unwired: 10 in, 1 out]
    n213 = Equal?(x=w337, y=WPI_DriverStationRobotMode2."Finish") -> (x = y?=w336:bool)
  }
